vi "Verify DLL.vi"(8 "error in":errorcluster) -> (0 "error out":errorcluster, 1 "DLL is Present":bool, 2 "path":path)   [LabVIEW 2009]
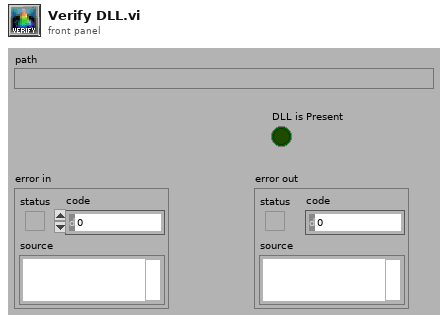
[diagram p1: front panel]
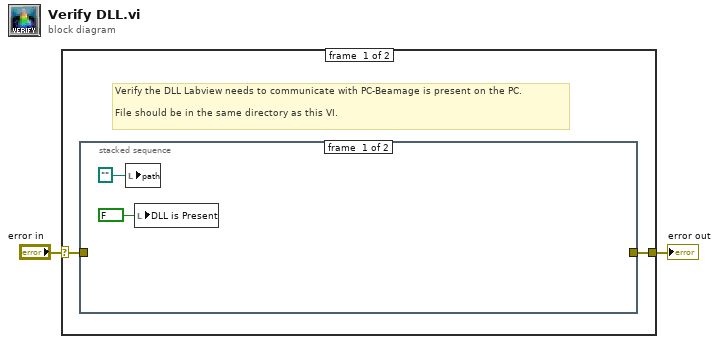
[diagram p0: block diagram]
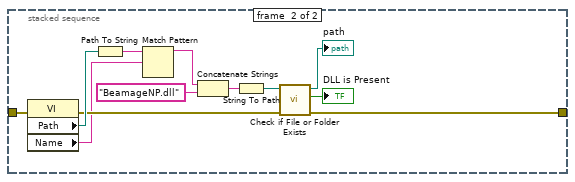
[diagram p2: hidden frame]
diagram:
  n1 = case shown="No Error" "error in" {
    selector: "error in" -> [w4 w19]
    tunnel: [w3 w19] -> w1
    frame #0 {
      # "Verify the DLL Labview needs to communicate with PC-Beamage is present on the PC.\n\nFile should be in the same directory as this VI."
      n2 = stacked-sequence {
        tunnel: w4 -> [_ w14]
        tunnel: [_ w12] -> w3
        frame #0 {
          n3 = local write "path"(path "") -> ()
          n4 = local write "DLL is Present"(FALSE ("file exists?")) -> ()
        }
        frame #1 {
          n5 = property class="VI"(error in=w14) -> (error out=w13:errorcluster, "Path"=w18:path, "Name"=w8:string)  [unwired: 1 in, 1 out]
          n6 = Path To String(path=w18) -> (string=w9:string)
          n7 = Match Pattern(string=w9, regular expression=w8) -> (before substring=w7:string)  [unwired: 1 in, 3 out]
          n8 = Concatenate Strings(w7, "BeamageNP.dll" ("string")) -> (w16:string)
          n9 = String To Path(string=w16) -> (path=w15:path)
          n10 = call <vilib>:"Check if File or Folder Exists.vi"("error in (no error)"=w13, "path"=w15) -> ("error out"=w12:errorcluster, "file or folder exists?"=→"DLL is Present":bool, "dup path"=→"path":path)  [unwired: 7 in]
        }
      }
    }
    frame #1 {
    }
  }
  "error out" <- w1
